vi "posicionled.vi"() -> ()   [LabVIEW 2016]
panel:
  in  "Stop Button":bool
  out "Boolean":bool
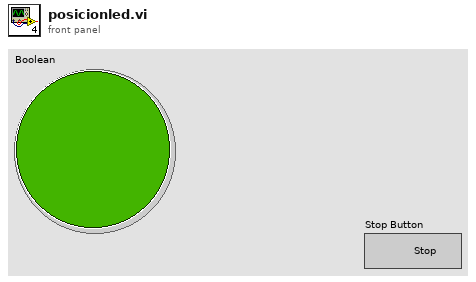
[diagram p1: front panel]
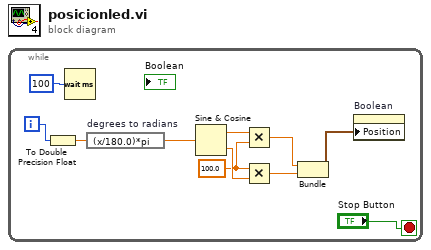
[diagram p0: block diagram]
diagram:
  n1 = while {
    i -> [w9]
    stop <- "Stop Button" stop-if-true
    w4 = 100.0 ("y")
    n2 = To Double Precision Float(number=w9) -> (double precision float=w8:dbl)
    n3 = Wait (ms)(milliseconds to wait=u32 100) -> ()  [unwired: 1 out]
    n4 = expression code="(x/180.0)*pi" "degrees to radians"(w8) -> (w7:dbl)
    n5 = Sine & Cosine(0:w7) -> (1:w6:dbl, 2:w5:dbl)
    n6 = Multiply(x=w6, y=w4) -> (x*y=w2:dbl)
    n7 = Multiply(x=w4, y=w5) -> (x*y=w3:dbl)
    n8 = Bundle(w2, w3) -> (w1:cluster{dbl, dbl})  [unwired: 1 in]
    n9 = property on="Boolean" class="Bool (strict)"("Position"=w1) -> ()  [unwired: 2 in, 2 out]
  }
